vi "divide.vi"(4 "State":i16, 5 "Time":dbl format="%.2f", 6 "Sensor Values":dbl[](array[numeric]), 7 "Set Points":dbl[](array[numeric])) -> (0 "required data":T1={"Set Point names"=["set point 1", "set point 2"], "required number of setpoints"=2, "required number of sensors"=0, "Sensor names"=[]}, 3 "output value":dbl)   [LabVIEW 2010]
panel:
  # "Enter the correct information for this control code in the required data structure below. Then make the current value default by right clicking on the border of the data structure. Select \"data operations\" and then select \"make current value default\". These values will be displayed by process controller."
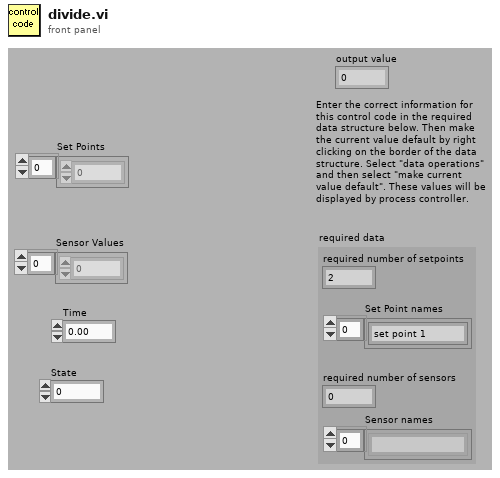
[diagram p1: front panel]
types:
  T1 = cluster{"Set Point names":string[], "required number of setpoints":u8, "required number of sensors":u8, "Sensor names":string[]}
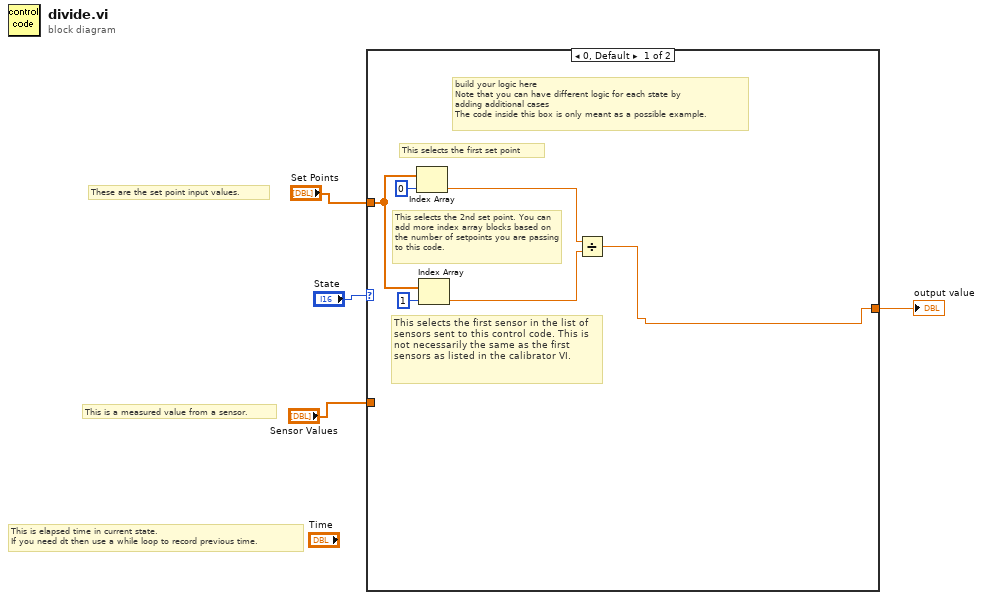
[diagram p0: block diagram]
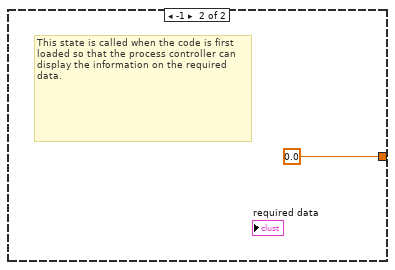
[diagram p2: hidden frame]
diagram:
  # "These are the set point input values."
  # "This is a measured value from a sensor."
  # "This is elapsed time in current state.\nIf you need dt then use a while loop to record previous time."
  n1 = case shown="0, Default" "State" {
    tunnel: [w5 0.0 ("fraction on")] -> w3
    tunnel: "Set Points" -> [w10 _]
    tunnel: "Sensor Values" -> [_ _]
    frame 0, Default {
      # "This selects the first sensor in the list of sensors sent to this control code. This is not necessarily the same as the first sensors as listed in the calibrator VI."
      # "This selects the 2nd set point. You can add more index array blocks based on the number of setpoints you are passing to this code."
      # "This selects the first set point"
      # "build your logic here\nNote that you can have different logic for each state by\nadding additional cases\nThe code inside this box is only meant as a possible example."
      n2 = Index Array(array=w10, index=0) -> (element=w7:dbl)
      n3 = Index Array(array=w10, index=1) -> (element=w6:dbl)
      n4 = Divide(x=w7, y=w6) -> (x/y=w5:dbl)
    }
    frame -1 {
      # "This state is called when the code is first loaded so that the process controller can display the information on the required data."
    }
  }
  "output value" <- w3
